vi "Read Deadzone.vi"(8 "error in (no error)":errorcluster, 11 "DriverXBoxController in":refnum<class "DriverXBoxController.lvclass">) -> (0 "error out":errorcluster, 2 "Deadzone":dbl=0.2, 3 "DriverXBoxController out":refnum<class "DriverXBoxController.lvclass">)   [LabVIEW 2013, in "DriverXBoxController.lvclass"]
uses:
  DriverXBoxController.lvclass
  DriverXBoxController.lvclass/DriverXBoxController.ctl
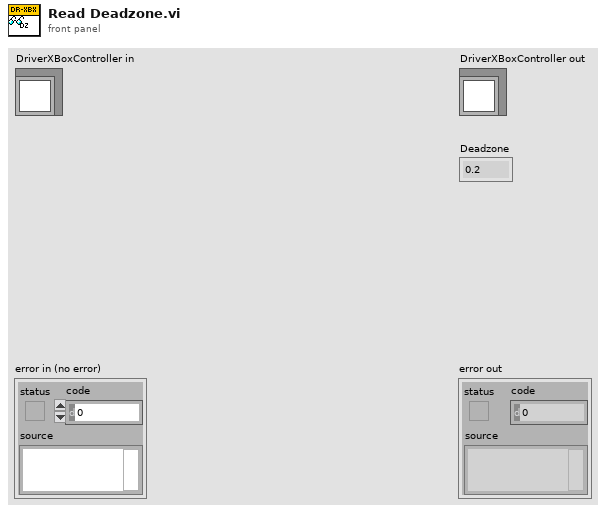
[diagram p1: front panel]
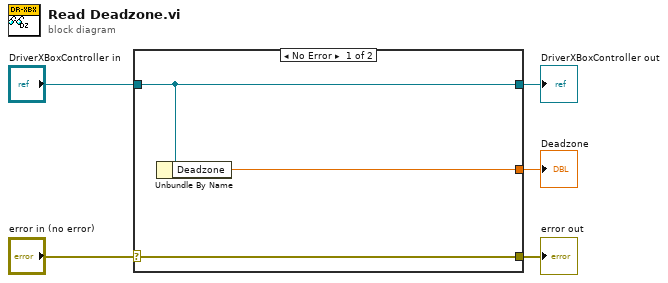
[diagram p0: block diagram]
diagram:
  n1 = case shown="No Error" "error in (no error)" {
    selector: "error in (no error)" -> [w8 w9]
    tunnel: [w8 w9] -> w4
    tunnel: [w7 w10] -> w2
    tunnel: "DriverXBoxController in" -> [w7 w10]
    tunnel: [w6 _] -> w1
    frame No Error {
      n2 = Unbundle By Name(w7) -> ("Deadzone"=w6:dbl)
    }
    frame Error {
    }
  }
  "error out" <- w4
  "DriverXBoxController out" <- w2
  "Deadzone" <- w1
